vi "Wait (SubVI).vi"(4 "error in":errorcluster, 12 "attente (ms)":u32) -> (24 "error out":errorcluster)   [LabVIEW 2017]
doc: "Add a soft wait througth the error.\nMade by Tanguy BOULARD\nTHALES FRANCE"
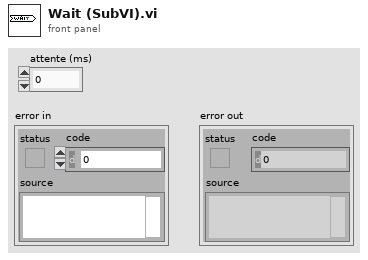
[diagram p1: front panel]
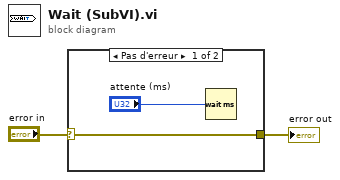
[diagram p0: block diagram]
diagram:
  n1 = case shown="Pas d'erreur" "error in" {
    selector: "error in" -> [w4 w5]
    tunnel: [w4 w5] -> w2
    frame No Error {
      n2 = Wait (ms)(milliseconds to wait="attente (ms)") -> ()  [unwired: 1 out]
    }
    frame Error {
    }
  }
  "error out" <- w2
